vi "Calculate_TargetOffset_Method2.vi"(9 "distance":dbl, 10 "skew":dbl, 11 "depth":dbl) -> (1 "max possible":dbl, 3 "target offset":dbl)   [LabVIEW 2019]
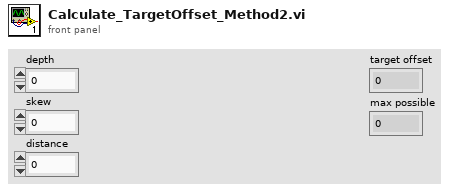
[diagram p1: front panel]
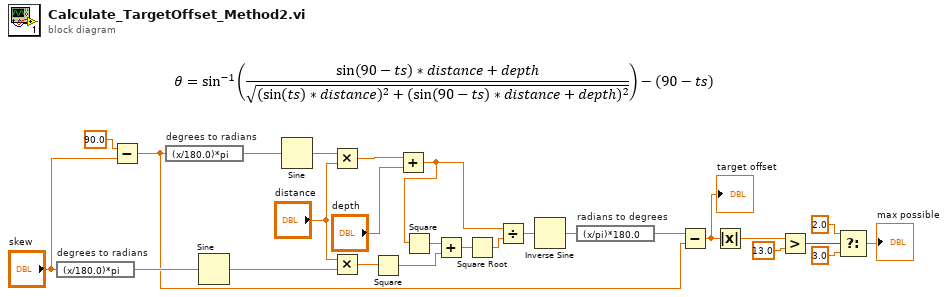
[diagram p0: block diagram]
diagram:
  n1 = expression code="(x/180.0)*pi" "degrees to radians"("skew") -> (w19:dbl)
  n2 = Subtract(x=90.0, y="skew") -> (x-y=w4:dbl)
  n3 = expression code="(x/180.0)*pi" "degrees to radians"(w4) -> (w20:dbl)
  n4 = Sine(x=w19) -> (sin(x)=w15:dbl)
  n5 = Sine(x=w20) -> (sin(x)=w17:dbl)
  n6 = Multiply(x=w17, y="distance") -> (x*y=w2:dbl)
  n7 = Multiply(x="distance", y=w15) -> (x*y=w13:dbl)
  n8 = Square(x=w13) -> (x^2=w11:dbl)
  n9 = Add(x=w2, y="depth") -> (x+y=w1:dbl)
  n10 = Square(x=w1) -> (x^2=w12:dbl)
  n11 = Add(x=w12, y=w11) -> (x+y=w10:dbl)
  n12 = Square Root(x=w10) -> (sqrt(x)=w9:dbl)
  n13 = Divide(x=w1, y=w9) -> (x/y=w8:dbl)
  n14 = Inverse Sine(1:w8) -> (0:w18:dbl)
  n15 = expression code="(x/pi)*180.0" "radians to degrees"(w18) -> (w7:dbl)
  n16 = Subtract(x=w7, y=w4) -> (x-y=w3:dbl)
  "target offset" <- w3
  n17 = Absolute Value(x=w3) -> (abs(x)=w26:dbl)
  n18 = Greater?(x=w26, y=13.0) -> (0:w24:bool)
  n19 = Select(t=2.0, s=w24, f=3.0) -> (s? t:f=→"max possible":dbl)
